vi "Main.vi"() -> ()   [LabVIEW 2019, in "Acquisition Example.lvlib"]
uses:
  Acquisition Example.lvlib
  Acquisition States.ctl
  Module Data.ctl
  Save Data.ctl
  Spectrometer/Module Data--cluster.ctl
  Spectrometer-LVClass/Abstract Spectrometer_class/Abstract Spectrometer.lvclass
  Camera/Module Data--cluster.ctl
  Camera/ROI--cluster.ctl
  Camera-LVClass/Picam_class/Picam.lvclass
  <vilib>/Analysis/1siggen.llb/Ramp Pattern by Samples.vi
  Camera/Camera.lvlib
  FileIO/FileIO.lvlib
  Spectrometer/Spectrometer.lvlib
  <vilib>/Analysis/NI_AALBase.lvlib
  Notification/Notification.lvlib
panel:
  in  "Comment":string
  in  "Measurement Name":string
  in  "Start":bool
  out "State":string
  out "Current Wavelength":dbl
  out "Waveform Graph":u16[](graph)
  in  "Wavelength Steps":u64
  in  "Wavelength End":dbl
  in  "Wavelength Start":dbl
  in  "Exposure Time":i64
  in  "Stop":bool
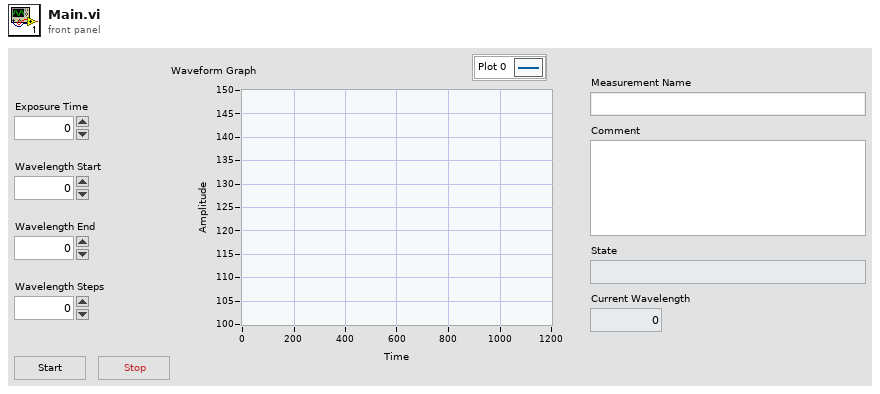
[diagram p1: front panel]
types:
  T1 = typedef "Acquisition Example.lvlib/Save Data.ctl" = cluster{"Acquisition":T2, "Spectrometer":T3, "Camera":T4}
  T2 = typedef "Acquisition Example.lvlib/Module Data.ctl" = cluster{"-File Path":path, "_Comment":string, "Iteration":u64, "-Initialized":bool}
  T3 = typedef "Spectrometer.lvlib/Module Data--cluster.ctl" = cluster{"Status":string, "-Abstract Spectrometer.lvclass":refnum<class "Abstract Spectrometer.lvclass">, "Device Data":cluster{"Wavelength":dbl, "Slit Width":dbl, "Grating ID":u32}}
  T4 = typedef "Camera.lvlib/Module Data--cluster.ctl" = cluster{"Status":string, "Image":u16[][], "Device Settings":cluster{"Accumulations":i64, "ROI":T5}, "-Picam Object":refnum<class "Picam.lvclass">}
  T5 = typedef "Camera.lvlib/ROI--cluster.ctl" = cluster{"_Horizontal":i32, "_Horizontal Width":i32, "_Horizontal Binning":i32, "_Vertical":i32, "_Vertical Width":i32, "_Vertical Binning":i32}
  T6 = typedef "Acquisition Example.lvlib/Acquisition States.ctl" = enum16{"Cleanup", "Initialize Dark Acquisition", "Set Spectrometer Wavelength", "Save Data", "Acquire Spectrum", "Initialize Acquisition", "Update Data", "Idle"}
  T7 = typedef "Spectrometer.lvlib/Set Wavelength (Reply Payload)--cluster.ctl" = cluster{"Wavelength":dbl, "Set Wavelength_error":errorcluster}
  T8 = typedef "Camera.lvlib/Get Image (Reply Payload)--cluster.ctl" = cluster{"Image":u16[][], "Get Image_error":errorcluster}
  T9 = typedef "FileIO.lvlib/Prepare File (Reply Payload)--cluster.ctl" = cluster{"success":bool, "file path":path, "Prepare File_error":errorcluster}
  T10 = typedef "Spectrometer.lvlib/Get Module Data (Reply Payload)--cluster.ctl" = cluster{"Spectrometer":T3, "Get Module Data_error":errorcluster}
  T11 = typedef "Camera.lvlib/Get Module Data (Reply Payload)--cluster.ctl" = cluster{"Camera":T4, "Get Module Data_error":errorcluster}
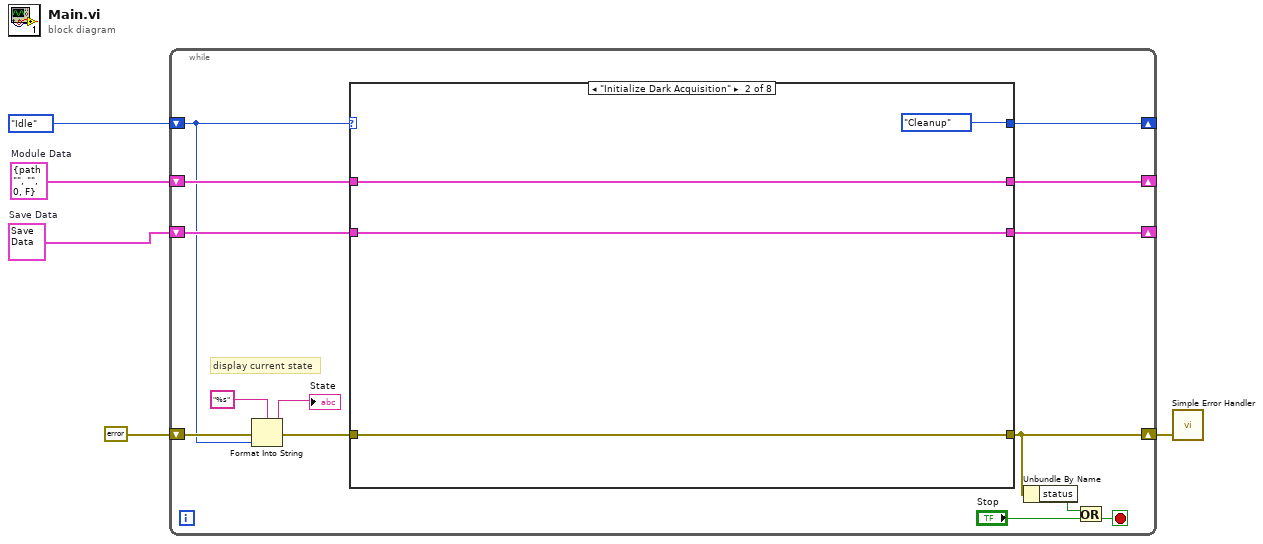
[diagram p0: block diagram]
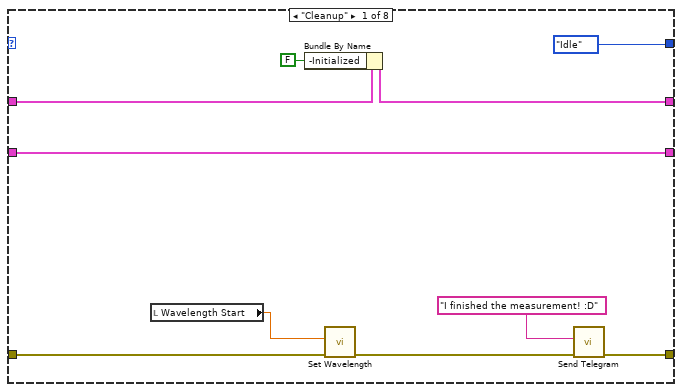
[diagram p2: hidden frame]
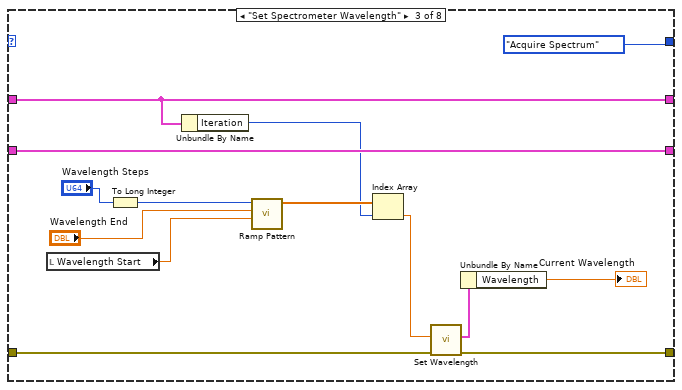
[diagram p3: hidden frame]
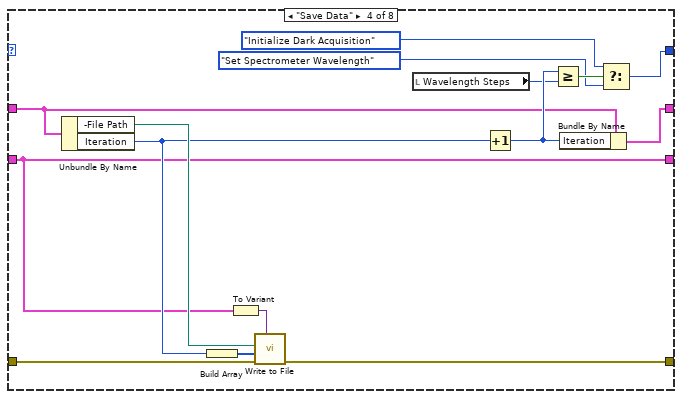
[diagram p4: hidden frame]
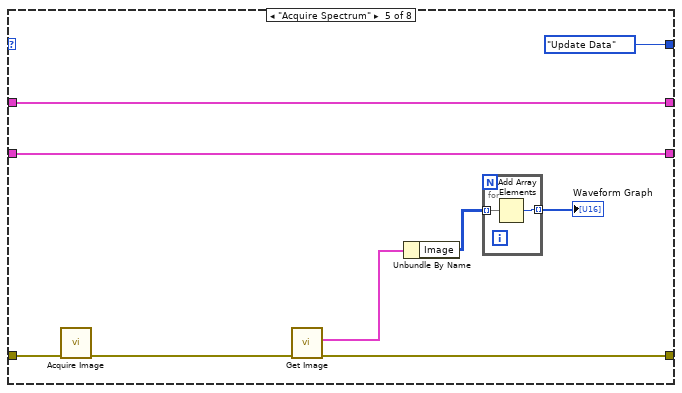
[diagram p5: hidden frame]
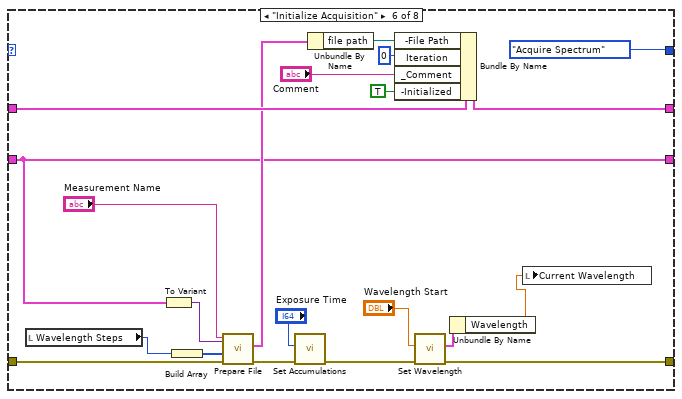
[diagram p6: hidden frame]
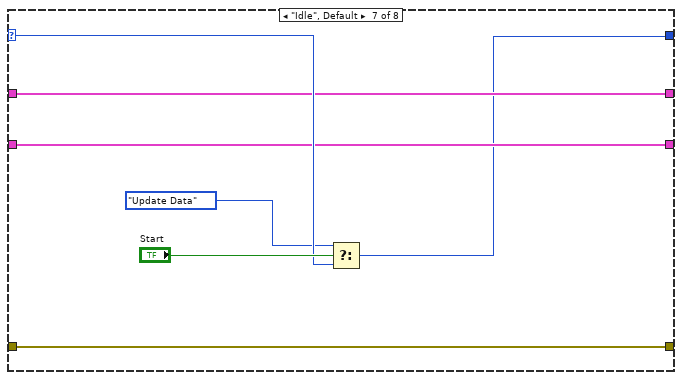
[diagram p7: hidden frame]
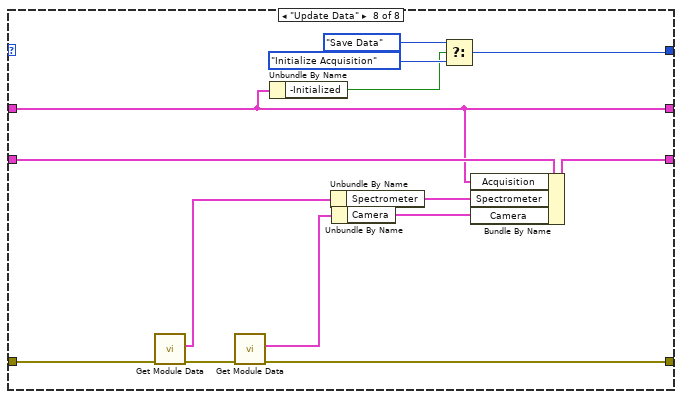
[diagram p8: hidden frame]
diagram:
  w2 = T1 {"Acquisition"={"-File Path"=path "", "_Comment"="", "Iteration"=0, "-Initialized"=FALSE}, "Spectrometer"={"Status"="", "-Abstract Spectrometer.lvclass"=refnum, "Device Data"={"Wavelength"=0.0, "Slit Width"=0.0, "Grating ID"=0}}, "Camera"={"Status"="", "Image"=[], "Device Settings"={"Accumulations"=0, "ROI"={"_Horizontal"=0, "_Horizontal Width"=0, "_Horizontal Binning"=0, "_Vertical"=0, "_Vertical Width"=0, "_Vertical Binning"=0}}, "-Picam Object"=refnum}}  # Save Data
  w3 = T2 {"-File Path"=path "", "_Comment"="", "Iteration"=0, "-Initialized"=FALSE}  # Module Data
  n1 = while {
    shift-right: [w16] -> w4
    shift-left: errorcluster {"status"=FALSE, "code"=0, "source"=""} ("error constant") -> [w18]
    shift-right: [w11] -> _
    shift-left: w3 -> [w12]
    shift-right: [w8] -> _
    shift-left: w2 -> [w9]
    shift-right: [w7] -> _
    shift-left: Acquisition_States."Idle" ("Enum") -> [w6]
    stop <- w17 stop-if-true
    # "display current state"
    n2 = Format Into String(format string="%s", error in=w18, w6) -> (resulting string=→"State":string, error out=w14:errorcluster)  [unwired: 1 in]
    n3 = case shown="\"Initialize Dark Acquisition\"" w6 {
      selector: w6 -> [_ _ _ _ _ _ w99 _]
      tunnel: w14 -> [w29 w32 w47 w62 w71 w94 w101 w115]
      tunnel: [w20 w32 w46 w61 w69 w87 w101 w113] -> w16
      tunnel: w12 -> [w26 w33 w36 w49 w65 w92 w98 w102]
      tunnel: [w24 w33 w36 w58 w65 w85 w98 w102] -> w11
      tunnel: w9 -> [w28 w31 w37 w48 w64 w81 w97 w114]
      tunnel: [w28 w31 w37 w48 w64 w81 w97 w111] -> w8
      tunnel: [Acquisition_States."Idle" ("Enum") Acquisition_States."Cleanup" ("Enum") Acquisition_States."Acquire Spectrum" ("Enum") w50 Acquisition_States."Update Data" ("Enum") Acquisition_States."Acquire Spectrum" ("Enum") w95 w107] -> w7
      frame "Cleanup" {
        n4 = local read "Wavelength Start"() -> (w27:dbl)
        n5 = Bundle By Name(cluster=w26, "-Initialized"=FALSE) -> (w24:T2)
        n6 = call "Set Wavelength.vi"("error in (no error)"=w29, "Wavelength"=w27) -> ("error out"=w22:errorcluster)  [unwired: 7 in, 2 out]
        n7 = call "Send Telegram.vi"("error in (no error)"=w22, "message"="I finished the measurement! :D") -> ("error out"=w20:errorcluster)  [unwired: 8 in]
      }
      frame "Initialize Dark Acquisition" {
      }
      frame "Set Spectrometer Wavelength" {
        n8 = local read "Wavelength Start"() -> (w42:dbl)
        n9 = To Long Integer(number="Wavelength Steps") -> (32bit integer=w44:i32)
        n10 = Unbundle By Name(w36) -> ("Iteration"=w35:u64)
        n11 = call-poly <vilib>:"Ramp Pattern.vi"("start"=w42, "end"="Wavelength End", "samples"=w44) -> ("Ramp Pattern"=w41:dbl[])  [unwired: 7 in, 1 out]
        n12 = Index Array(array=w41, index=w35) -> (element=w40:dbl)
        n13 = call "Set Wavelength.vi"("error in (no error)"=w47, "Wavelength"=w40) -> ("error out"=w46:errorcluster, "Reply Payload"=w39:T7)  [unwired: 7 in, 1 out]
        n14 = Unbundle By Name(w39) -> ("Wavelength"=→"Current Wavelength":dbl)
      }
      frame "Save Data" {
        n15 = Unbundle By Name(w49) -> ("-File Path"=w59:path, "Iteration"=w54:u64)
        n16 = Build Array(w54) -> (w53:u64[])
        n17 = To Variant(anything=w48) -> (Variant=w60:variant)
        n18 = call "Write to File.vi"("data"=w60, "error in (no error)"=w62, "indices"=w53, "file path"=w59) -> ("error out"=w61:errorcluster)  [unwired: 5 in, 2 out]
        n19 = local read "Wavelength Steps"() -> (w56:u64)
        n20 = Increment(x=w54) -> (x+1=w57:u64)
        n21 = Greater Or Equal?(x=w57, y=w56) -> (x >= y?=w55:bool)
        n22 = Bundle By Name(cluster=w49, "Iteration"=w57) -> (w58:T2)
        n23 = Select(t=Acquisition_States."Initialize Dark Acquisition" ("Enum"), s=w55, f=Acquisition_States."Set Spectrometer Wavelength" ("Enum")) -> (s? t:f=w50:T6)
      }
      frame "Acquire Spectrum" {
        n24 = call "Acquire Image.vi"("error in (no error)"=w71) -> ("error out"=w70:errorcluster)  [unwired: 10 in]
        n25 = call "Get Image.vi"("error in (no error)"=w70) -> ("error out"=w69:errorcluster, "Reply Payload"=w68:T8)  [unwired: 8 in, 1 out]
        n26 = Unbundle By Name(w68) -> ("Image"=w67:u16[][])
        n27 = for {
          tunnel: w67 -> [w73] mode=indexing
          tunnel: [w72] -> w66 mode=indexing
          n28 = Add Array Elements(numeric array=w73) -> (sum=w72:u16)
        }
        "Waveform Graph" <- w66
      }
      frame "Initialize Acquisition" {
        n29 = local read "Wavelength Steps"() -> (w79:u64)
        n30 = To Variant(anything=w81) -> (Variant=w91:variant)
        n31 = Build Array(w79) -> (w78:u64[])
        n32 = call "Prepare File.vi"("data"=w91, "error in (no error)"=w94, "dims"=w78, "Measurement Name"="Measurement Name") -> ("error out"=w93:errorcluster, "Reply Payload"=w86:T9)  [unwired: 5 in, 1 out]
        n33 = call "Set Accumulations.vi"("error in (no error)"=w93, "Accumulations"="Exposure Time") -> ("error out"=w89:errorcluster)  [unwired: 7 in, 2 out]
        n34 = Unbundle By Name(w86) -> ("file path"=w84:path)
        n35 = Bundle By Name(cluster=w92, "-File Path"=w84, "Iteration"=u64 0 ("-Iteration"), "_Comment"="Comment", "-Initialized"=TRUE) -> (w85:T2)
        n36 = call "Set Wavelength.vi"("error in (no error)"=w89, "Wavelength"="Wavelength Start") -> ("error out"=w87:errorcluster, "Reply Payload"=w83:T7)  [unwired: 7 in, 1 out]
        n37 = Unbundle By Name(w83) -> ("Wavelength"=w82:dbl)
        n38 = local write "Current Wavelength"(w82) -> ()
      }
      frame "Idle", Default {
        n39 = Select(t=Acquisition_States."Update Data" ("Enum"), s="Start", f=w99) -> (s? t:f=w95:T6)
      }
      frame "Update Data" {
        n40 = call "Get Module Data.vi"("error in (no error)"=w115) -> ("error out"=w112:errorcluster, "Reply Payload"=w109:T10)  [unwired: 8 in, 1 out]
        n41 = call "Get Module Data.vi"("error in (no error)"=w112) -> ("error out"=w113:errorcluster, "Reply Payload"=w110:T11)  [unwired: 8 in, 1 out]
        n42 = Unbundle By Name(w102) -> ("-Initialized"=w105:bool)
        n43 = Unbundle By Name(w109) -> ("Spectrometer"=w103:T3)
        n44 = Unbundle By Name(w110) -> ("Camera"=w104:T4)
        n45 = Select(t=Acquisition_States."Save Data", s=w105, f=Acquisition_States."Initialize Acquisition" ("Enum")) -> (s? t:f=w107:T6)
        n46 = Bundle By Name(cluster=w114, "Acquisition"=w102, "Spectrometer"=w103, "Camera"=w104) -> (w111:T1)
      }
    }
    n47 = Unbundle By Name(w16) -> ("status"=w15:bool)
    n48 = Or(x=w15, y="Stop") -> (x .or. y?=w17:bool)
  }
  n49 = call <vilib>:"Simple Error Handler.vi"("error in (no error)"=w4) -> ()  [unwired: 4 in, 5 out]
